vi "dfd_FLP Lattice One Multiplier Section.vi"(3 "k(m)":dbl format="%.2f", 4 "w(m-1)":dbl format="%.2f", 5 "x(m)":dbl format="%.2f") -> (0 "u(m)":dbl, 1 "w(m)":dbl format="%.2f", 2 "x(m-1)":dbl format="%.2f")   [LabVIEW 2017, in "NI_DigFilter_FXP.lvlib"]
uses:
  <vilib>/addons/Digital Filter Design/NI_DigFilter_FXP.lvlib
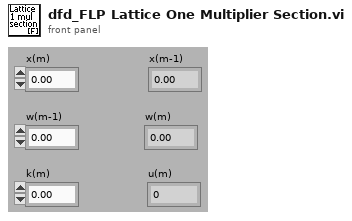
[diagram p1: front panel]
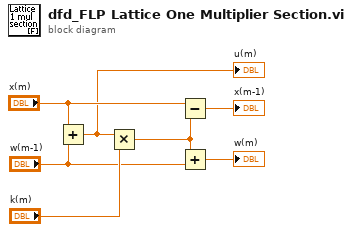
[diagram p0: block diagram]
diagram:
  n1 = Add(x="x(m)", y="w(m-1)") -> (x+y=w1:dbl)
  "u(m)" <- w1
  n2 = Multiply(x=w1, y="k(m)") -> (x*y=w4:dbl)
  n3 = Subtract(x="x(m)", y=w4) -> (x-y=→"x(m-1)":dbl)
  n4 = Add(x=w4, y="w(m-1)") -> (x+y=→"w(m)":dbl)
